vi "ArmPathPlanner.vi"(0 "StartPoint":T5, 1 "EndPoint":T5, 2 "PathPointSpacing (in)":dbl, 3 "MinArmLength":dbl, 4 "MaxArmLength":dbl, 5 "AvoidancePolygon":T4, 7 "MotionProfileGeneratorParameters":T3={"Trajectory Point Interval (ms)"=10, "Maximum Travel Speed (rpm)"=0.0, "Velocity Ramp Time (ms)"=0.0, "Acceleration Ramp Time (ms)"=1.0} {"Acceleration Ramp Time (ms)" min=1.0; "Velocity Ramp Time (ms)" min=1.0; "Maximum Travel Speed (rpm)" min=0.0; "Trajectory Point Interval (ms)" items=["TrajectoryDuration_0ms"=0, "TrajectoryDuration_5ms"=5, "TrajectoryDuration_10ms"=10, "TrajectoryDuration_20ms"=20, "TrajectoryDuration_30ms"=30, "TrajectoryDuration_40ms"=40, "TrajectoryDuration_50ms"=50, "TrajectoryDuration_100ms"=100]}) -> (14 "Path":T6[](array[typedef]), 15 "RotatePath":T1[](array[typedef]) {"Time (ms)" items=["TrajectoryDuration_0ms"=0, "TrajectoryDuration_5ms"=5, "TrajectoryDuration_10ms"=10, "TrajectoryDuration_20ms"=20, "TrajectoryDuration_30ms"=30, "TrajectoryDuration_40ms"=40, "TrajectoryDuration_50ms"=50, "TrajectoryDuration_100ms"=100]}, 16 "ExtendPath":T1[](array[typedef]) {"Time (ms)" items=["TrajectoryDuration_0ms"=0, "TrajectoryDuration_5ms"=5, "TrajectoryDuration_10ms"=10, "TrajectoryDuration_20ms"=20, "TrajectoryDuration_30ms"=30, "TrajectoryDuration_40ms"=40, "TrajectoryDuration_50ms"=50, "TrajectoryDuration_100ms"=100]}, 19 "PathLength (in)":dbl)   [LabVIEW 2017]
uses:
  TypeDefs/ArmCoordinate.ctl
  General/PathPlanning/TypeDefs/Point2D.ctl
  General/PathPlanning/TypeDefs/Polygon2D.ctl
  General/MotionProfiling/TypeDefs/MotionProfileGeneratorParams.ctl
  <vilib>/Rock Robotics/WPI/ThirdParty/Phoenix-LabVIEW/Motor Controller/Controls/CTRE_Phoenix_MotorControl_TrajectoryPointTimeDur.ctl
  General/MotionProfiling/TypeDefs/TrajectoryPoint.ctl
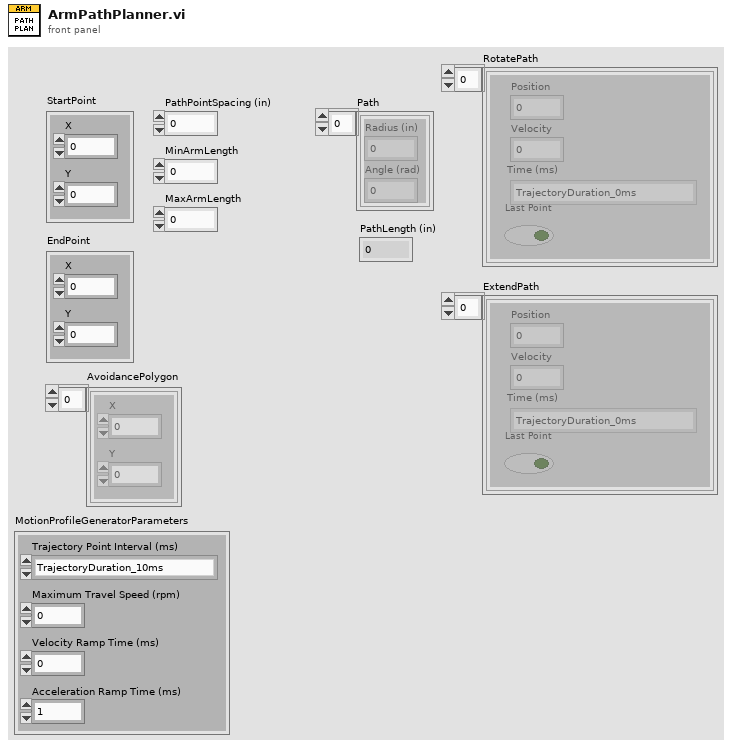
[diagram p1: front panel]
types:
  T1 = typedef "TrajectoryPoint.ctl" = cluster{"Position ":dbl, "Velocity ":dbl, "Time (ms)":T2, "Last Point":bool}
  T2 = typedef "CTRE_Phoenix_MotorControl_TrajectoryPointTimeDur.ctl" = i32
  T3 = typedef "MotionProfileGeneratorParams.ctl" = cluster{"Trajectory Point Interval (ms)":T2, "Maximum Travel Speed (rpm)":dbl, "Velocity Ramp Time (ms)":dbl, "Acceleration Ramp Time (ms)":dbl}
  T4 = typedef "Polygon2D.ctl" = T5[]
  T5 = typedef "Point2D.ctl" = cluster{"X":dbl, "Y":dbl}
  T6 = typedef "ArmCoordinate.ctl" = cluster{"Radius (in)":dbl, "Angle (rad)":dbl}
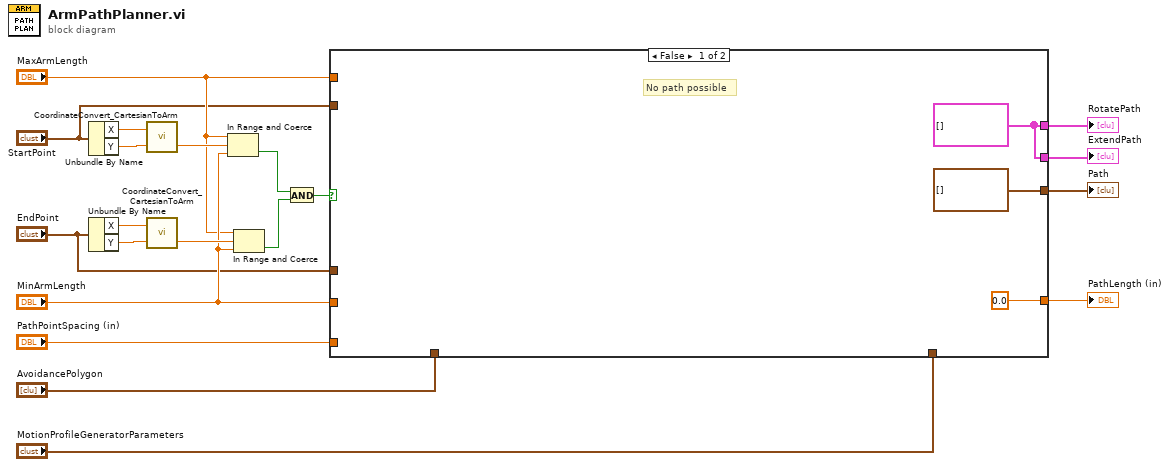
[diagram p0: block diagram]
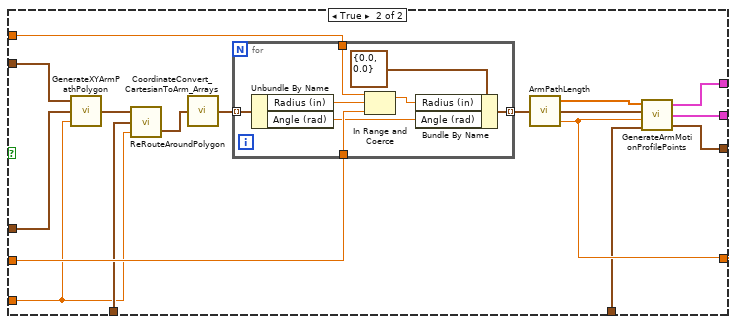
[diagram p2: hidden frame]
diagram:
  n1 = Unbundle By Name("StartPoint") -> ("X"=w10:dbl, "Y"=w9:dbl)
  n2 = Unbundle By Name("EndPoint") -> ("X"=w8:dbl, "Y"=w7:dbl)
  n3 = call "CoordinateConvert_CartesianToArm.vi"("Y (in)"=w9, "X (in)"=w10) -> ("Radius (in)"=w20:dbl)  [unwired: 1 out]
  n4 = call "CoordinateConvert_CartesianToArm.vi"("Y (in)"=w7, "X (in)"=w8) -> ("Radius (in)"=w19:dbl)  [unwired: 1 out]
  n5 = In Range and Coerce(upper limit="MaxArmLength", x=w20, lower limit="MinArmLength") -> (In Range?=w18:bool)  [unwired: 1 out]
  n6 = In Range and Coerce(upper limit="MaxArmLength", x=w19, lower limit="MinArmLength") -> (In Range?=w17:bool)  [unwired: 1 out]
  n7 = And(x=w18, y=w17) -> (x .and. y?=w16:bool)
  n8 = case shown="False" w16 {
    tunnel: [T6[] [] ("ArmPathOut") w26] -> w11
    tunnel: [0.0 w28] -> w15
    tunnel: "MinArmLength" -> [_ w39]
    tunnel: "MaxArmLength" -> [_ w40]
    tunnel: "PathPointSpacing (in)" -> [_ w32]
    tunnel: "StartPoint" -> [_ w38]
    tunnel: "EndPoint" -> [_ w37]
    tunnel: "AvoidancePolygon" -> [_ w33]
    tunnel: "MotionProfileGeneratorParameters" -> [_ w27]
    tunnel: [w21 w25] -> w2
    tunnel: [w21 w24] -> w1
    frame False {
      w21 = T1[] [] ("ExtendPath")
      # "No path possible"
    }
    frame True {
      n9 = call "GenerateXYArmPathPolygon.vi"("PointSpacing (in)"=w32, "EndPoint"=w37, "StartPoint"=w38) -> ("XYPathPoints"=w34:T5[])
      n10 = call "ReRouteAroundPolygon.vi"("Desired Point Spacing (in)"=w32, "AvoidancePolygon"=w33, "InputPath"=w34) -> ("OutputPath"=w31:T5[])  [unwired: 1 out]
      n11 = call "CoordinateConvert_CartesianToArm_Arrays.vi"("XYPoints"=w31) -> ("ArmCoordinates"=w36:T6[])
      n12 = for {
        tunnel: w40 -> [w48]
        tunnel: w39 -> [w47]
        tunnel: w36 -> [w46] mode=indexing
        tunnel: [w41] -> w35 mode=indexing
        n13 = Unbundle By Name(w46) -> ("Radius (in)"=w45:dbl, "Angle (rad)"=w44:dbl)
        n14 = In Range and Coerce(upper limit=w48, x=w45, lower limit=w47) -> (coerced(x)=w43:dbl)  [unwired: 1 out]
        n15 = Bundle By Name(cluster=T6 {"Radius (in)"=0.0, "Angle (rad)"=0.0} ("Point"), "Radius (in)"=w43, "Angle (rad)"=w44) -> (w41:T6)
      }
      n16 = call "ArmPathLength.vi"("ArmPathIn"=w35) -> ("Path Length"=w28:dbl, "ArmPathOut"=w29:T6[], "IndexedPathLength"=w30:dbl[])  [unwired: 2 in]
      n17 = call "GenerateArmMotionProfilePoints.vi"("MotionProfileGeneratorParameters"=w27, "PathDistance"=w28, "ArmPathIn"=w29, "IndexedPathLength"=w30) -> ("ArmPathOut"=w26:T6[], "ExtendPath"=w24:T1[], "RotatePath"=w25:T1[])
    }
  }
  "PathLength (in)" <- w15
  "Path" <- w11
  "RotatePath" <- w2
  "ExtendPath" <- w1
